vi "RT testbead.vi"() -> ()   [LabVIEW 2010]
uses:
  <vilib>/Instr/_visa.llb/VISA Configure Serial Port (Instr).vi
  behaviors/driveable path/drivable paths global.vi
  Deleteme/line driveable paths global.vi
panel:
  out "XY Graph":cluster{"Y":dbl[], "Y":dbl[]}[](graph)
  out "driveable path lengths (lines)":u16[](array[numeric])
  out "Serial Settings:Number of Bytes at Serial Port":u32
  in  "stop":bool
  out "read buffer":string
  in  "VISA resource name":refnum<visa-resource-name>
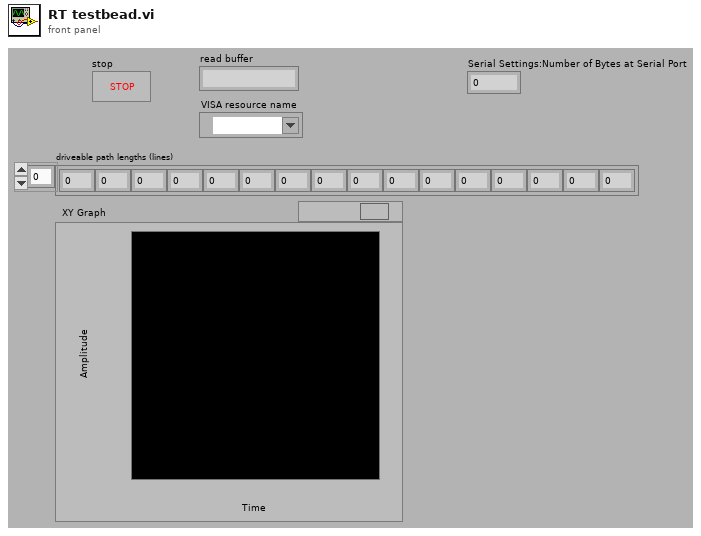
[diagram p1: front panel]
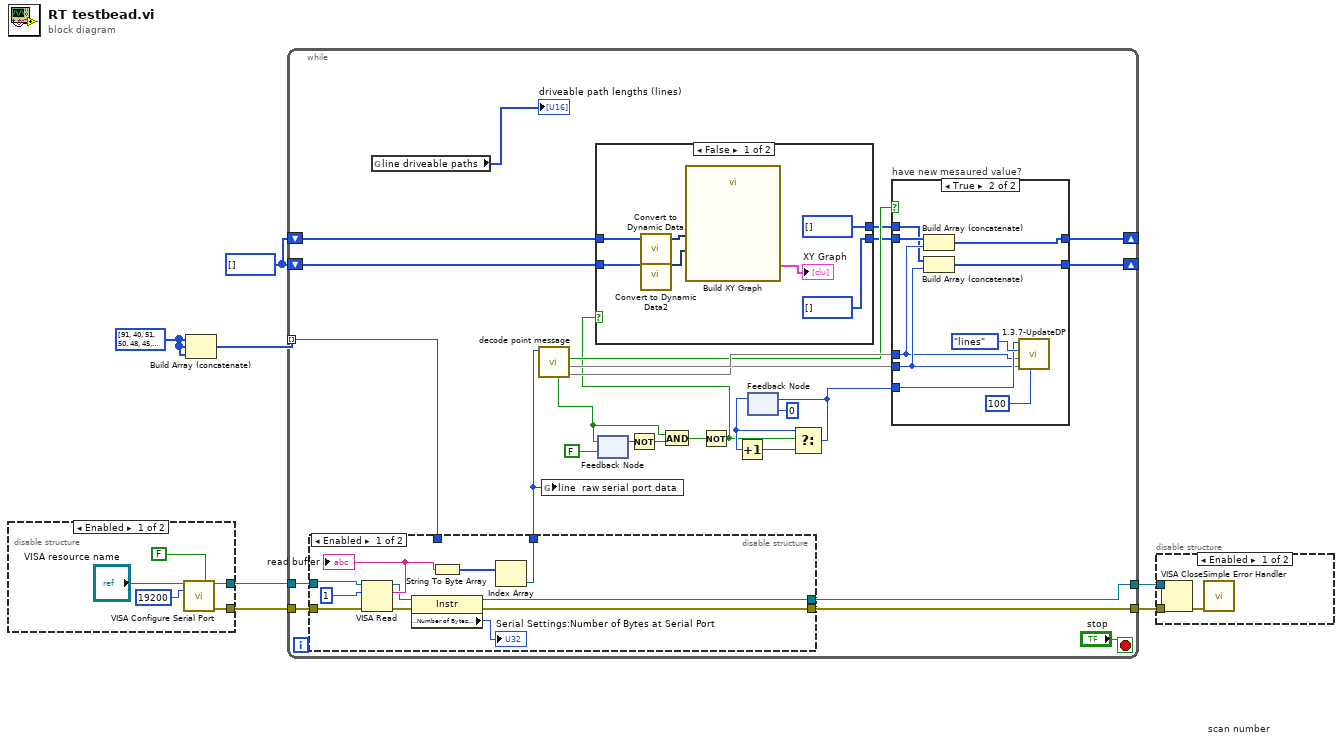
[diagram p0: block diagram]
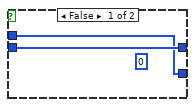
[diagram p6: hidden frame]
diagram:
  w1 = u8[] [91, 40, 51, 50, 48, 45, 44, 55, 54, 48, 48, 41, 40, 49, 50, 48, 45, 44, 55, 54, 48, 48, 41, 40, 57, 49, 48, 45, 44, 55, 54, 48, 48, 41, 40, 51, 50, 48, 45, 44, 53, 54, 48, 48, 41, 40, 49, 50, 48, 45, 44, 53, 54, 48, 48, 41, 40, 57, 49, 48, 45, 44, 53, 54, 48, 48, 41, 40, 50, 48, 48, 48, 44, 53, 54, 48, 48, 41, 40, 53, 48, 48, 48, 44, 53, 54, 48, 48, 41, 40, 51, 50, 48, 45, 44, 51, 54, 48, 48, 41, 40, 49, 50, 48, 45, 44, 51, 54, 48, 48, 41, 40, 57, 49, 48, 45, 44, 51, 54, 48, 48, 41, 40, 50, 48, 48, 48, 44, 51, 54, 48, 48, 41, 40, 53, 48, 48, 48, 44, 51, 54, 48, 48, 41, 40, 55, 48, 48, 48, 44, 51, 54, 48, 48, 41, 40, 51, 50, 48, 45, 44, 48, 54, 48, 48, 41, 40, 49, 50, 48, 45, 44, 48, 54, 48, 48, 41, 40, 50, 48, 48, 48, 44, 48, 54, 48, 48, 41, 40, 53, 48, 48, 48, 44, 48, 54, 48, 48, 41, 40, 55, 48, 48, 48, 44, 48, 54, 48, 48, 41, 40, 50, 48, 48, 48, 44, 56, 53, 48, 48, 41, 40, 53, 48, 48, 48, 44, 56, 53, 48, 48, 41, 40, 55, 48, 48, 48, 44, 56, 53, 48, 48, 41, 93] ("vision points message")
  w3 = i16[] []
  n1 = disable-structure shown="Enabled" {
    disable-tunnel: [w9 _] -> w7
    disable-tunnel: [w8 _] -> w6
    frame Enabled {
      n2 = call-poly "VISA Configure Serial Port"("VISA resource name"="VISA resource name", "Enable Termination\nChar (T)"=FALSE ("Enable Termination\nChar (T)"), "baud rate (9600)"=u32 19200) -> ("VISA resource name out"=w9:refnum<visa-resource-name>, "error out"=w8:errorcluster)  [unwired: 11 in]
    }
    frame Disabled {
    }
  }
  n3 = Build Array (concatenate)(w1, w1, w1) -> (w2:u8[])
  n4 = while {
    tunnel: w7 -> [w39]
    tunnel: w6 -> [w38]
    tunnel: [w33] -> w5
    tunnel: [w32] -> w4
    shift-right: [w30] -> _
    shift-left: w3 -> [w27]
    shift-right: [w29] -> _
    shift-left: w3 -> [w28]
    tunnel: w2 -> [w14] mode=indexing
    stop <- "stop" stop-if-true
    n5 = disable-structure shown="Enabled" {
      disable-tunnel: w39 -> [w50 _]
      disable-tunnel: w38 -> [w49 _]
      disable-tunnel: [w45 w51] -> w34
      disable-tunnel: [w43 _] -> w33
      disable-tunnel: [w41 _] -> w32
      disable-tunnel: w14 -> [_ w51]
      frame Enabled {
        n6 = VISA Read(VISA resource name=w50, byte count=u32 1, error in (no error)=w49) -> (VISA resource name out=w44:refnum<visa-resource-name>, read buffer=w47:string, error out=w42:errorcluster)  [unwired: 1 out]
        "read buffer" <- w47
        n7 = property class="Instr"(reference=w44, error in=w42) -> (reference out=w43:refnum<visa-resource-name>, error out=w41:errorcluster, "Serial Settings:Number of Bytes at Serial Port"=→"Serial Settings:Number of Bytes at Serial Port":u32)
        n8 = String To Byte Array(string=w47) -> (unsigned byte array=w46:u8[])
        n9 = Index Array(array=w46) -> (element=w45:u8)  [unwired: 1 in]
      }
      frame Disabled {
      }
    }
    n10 = global read "line driveable paths global.vi" "line driveable paths"() -> (→"driveable path lengths (lines)":u16[])
    n11 = call "decode point message.vi"("input stream"=w34) -> (0:w35, 1:w36, "new y"=w31:bool, "waiting for new message"=w16:bool)  [unwired: 5 in, 2 out]
    n12 = global write "drivable paths global.vi" "line  raw serial port data"(w34) -> ()
    n13 = feedback-in #1(w16) -> ()
    n14 = feedback #1(FALSE) -> (w22:bool)
    n15 = Not(x=w22) -> (.not. x?=w24:bool)
    n16 = And(x=w16, y=w24) -> (x .and. y?=w23:bool)
    n17 = Not(x=w23) -> (.not. x?=w15:bool)
    n18 = case shown="False" w15 {
      tunnel: w28 -> [w55 w60]
      tunnel: w27 -> [w53 w59]
      tunnel: [i16[] [] w60] -> w26
      tunnel: [i16[] [] w59] -> w25
      frame False {
        n19 = call "Convert to Dynamic Data"("Array"=w55) -> ("Dynamic Data Type"=w54:dynamicdata)  [unwired: 3 in]
        n20 = call "Convert to Dynamic Data2"("Array"=w53) -> ("Dynamic Data Type"=w52:dynamicdata)  [unwired: 3 in]
        n21 = call "Build XY Graph"("Y Input"=w52, "X Input"=w54) -> ("XY Graph"=→"XY Graph":cluster{"Y":dbl[], "Y":dbl[]}[])  [unwired: 8 in, 1 out]
      }
      frame True {
      }
    }
    n22 = feedback #2 "scan number"(u8 0 ("y")) -> (w20:u8)
    n23 = Increment(x=w20) -> (x+1=w19:u8)
    n24 = Select(t=w20, s=w15, f=w19) -> (s? t:f=w17:u8)
    n25 = feedback-in #2(w17) -> ()
    n26 = case "have new mesaured value?" shown="True" w31 {
      tunnel: w36 -> [_ w68]
      tunnel: w35 -> [_ w69]
      tunnel: w17 -> [_ w70]
      tunnel: [w61 w67] -> w30
      tunnel: [w62 w66] -> w29
      tunnel: w26 -> [w62 w65]
      tunnel: w25 -> [w61 w64]
      frame False {
        (unwired) u8 0 ("y")
      }
      frame True {
        n27 = Build Array (concatenate)(w65, w68) -> (w66:i16[])
        n28 = Build Array (concatenate)(w64, w69) -> (w67:i16[])
        n29 = call "1.3.7-UpdateDP.vi"("allowed proximity squared"=i16 100, "Robot Y"=w69, "Robot X"=w68, "update lines or objects"=enum16{"lines", "obstacles"}."lines", "Scan Number"=w70) -> ()  [unwired: 7 in]
      }
    }
  }
  n30 = disable-structure shown="Enabled" {
    disable-tunnel: w5 -> [w73 _]
    disable-tunnel: w4 -> [w72 _]
    frame Enabled {
      n31 = VISA Close(VISA resource name=w73, error in (no error)=w72) -> (error out=w74:errorcluster)
      n32 = call <vilib>:"Simple Error Handler.vi"("error in (no error)"=w74) -> ()  [unwired: 4 in, 5 out]
    }
    frame Disabled {
    }
  }
